vi "Initialize Qeue.vi"(8 "error in (no error)":errorcluster, 11 "TCS in":refnum<class "TCS.lvclass">) -> (0 "error out":errorcluster, 3 "TCS out":refnum<class "TCS.lvclass">)   [LabVIEW 2018, in "TCS.lvclass"]
uses:
  TCS.lvclass
  TCS.lvclass/TCS.ctl
  RxTx/RxTx.lvclass
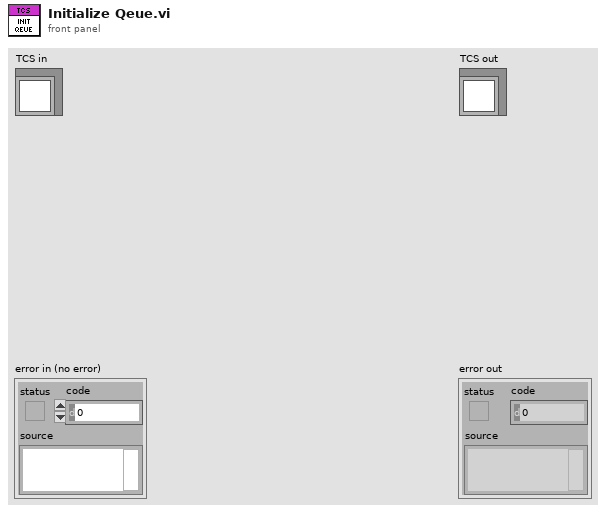
[diagram p1: front panel]
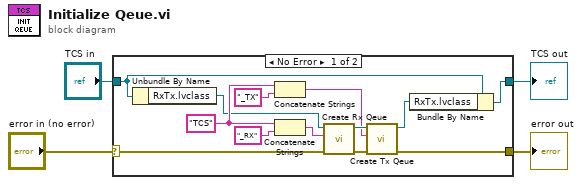
[diagram p0: block diagram]
diagram:
  n1 = case shown="No Error" "error in (no error)" {
    selector: "error in (no error)" -> [w12 w19]
    tunnel: [w9 w19] -> w2
    tunnel: [w16 w18] -> w1
    tunnel: "TCS in" -> [w17 w18]
    frame No Error {
      w13 = "TCS"
      n2 = Unbundle By Name(w17) -> ("RxTx.lvclass"=w11:refnum<class "RxTx.lvclass">)
      n3 = Concatenate Strings(w13, "_TX") -> (w5:string)
      n4 = Concatenate Strings(w13, "_RX") -> (w10:string)
      n5 = call "Create Rx Qeue.vi"("error in (no error)"=w12, "Reader Name"=w10, "RxTx in"=w11) -> ("error out"=w6:errorcluster, "RxTx out"=w7:refnum<class "RxTx.lvclass">)  [unwired: 7 in]
      n6 = call "Create Tx Qeue.vi"("error in (no error)"=w6, "Writer Name"=w5, "RxTx in"=w7) -> ("error out"=w9:errorcluster, "RxTx out"=w8:refnum<class "RxTx.lvclass">)  [unwired: 7 in]
      n7 = Bundle By Name(cluster=w17, "RxTx.lvclass"=w8) -> (w16:refnum<class "TCS.lvclass">)
    }
    frame Error {
    }
  }
  "error out" <- w2
  "TCS out" <- w1
